vi "Pre Launch Init.vi"(11 "Measure Object in":refnum<class "Template Module.lvclass">) -> (0 "error out":errorcluster, 3 "Measure Object out":refnum<class "Template Module.lvclass">)   [LabVIEW 2019, in "Template Module.lvclass"]
doc: "(<B>Filename</B>: Actor Framework.lvlib:Actor.lvclass:Pre Launch Init.vi)\n\nDefines behavior that occurs after the Launch Nested Actor method is invoked but before the actor's Actor Core method begins running.\n\nBy default, this method does nothing. A descendant class may override it to define behavior."
uses:
  Template Module.lvclass
  Template Module.lvclass/Template Module.ctl
  <vilib>/ActorFramework/Actor/Actor.lvclass
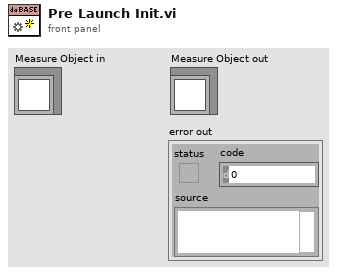
[diagram p1: front panel]
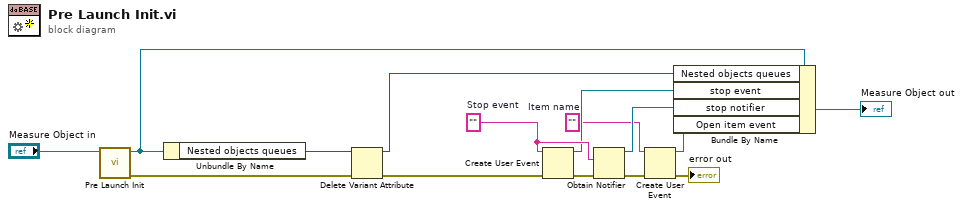
[diagram p0: block diagram]
diagram:
  w7 = ""  # Item name
  w14 = ""  # Stop event
  n1 = call-parent "Pre Launch Init.vi"("Actor in"="Measure Object in") -> ("error out"=w3:errorcluster, "Actor out"=w5:refnum<class "Template Module.lvclass">)  [unwired: 9 in]
  n2 = Unbundle By Name(w5) -> ("Nested objects queues"=w4:variant)
  n3 = Delete Variant Attribute(4:w3, 7:w4) -> (0:w2:errorcluster, 3:w1:variant)  [unwired: 1 in, 1 out]
  n4 = Create User Event(user event datatype=w14, error in=w2) -> (user event=w11:refnum<user-event>, error out=w13:errorcluster)
  n5 = Obtain Notifier(notification data type=w14, error in (no error)=w13) -> (notifier out=w10:refnum<notifier>, error out=w9:errorcluster)  [unwired: 2 in, 1 out]
  n6 = Create User Event(user event datatype=w7, error in=w9) -> (user event=w6:refnum<user-event>, error out=→"error out":errorcluster)
  n7 = Bundle By Name(cluster=w5, "Nested objects queues"=w1, "stop event"=w11, "stop notifier"=w10, "Open item event"=w6) -> (→"Measure Object out":refnum<class "Template Module.lvclass">)
